vi "Cmd.ReadProgram.vi"(6 "Timeout [ms] (1000)":i32=1000, 8 "error in":errorcluster, 11 "cID in":refnum<k5>) -> (0 "error out":errorcluster, 1 "ProgramNumber":u16, 2 "SDCard":u8, 3 "cID out":refnum<k5>)   [LabVIEW 2016]
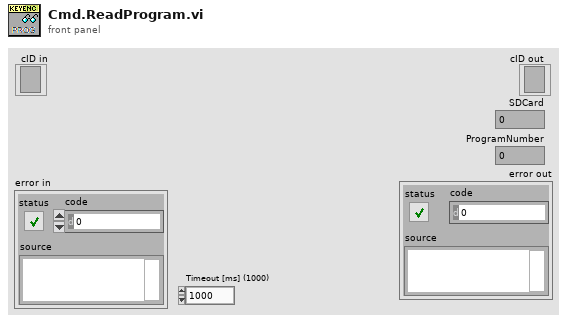
[diagram p1: front panel]
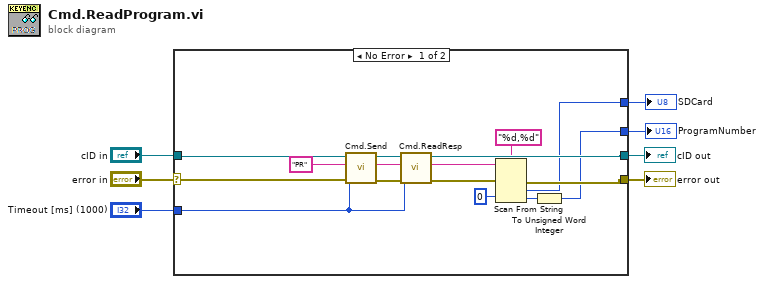
[diagram p0: block diagram]
diagram:
  n1 = case shown="No Error" "error in" {
    selector: "error in" -> [w21 w23]
    tunnel: "Timeout [ms] (1000)" -> [w18 _]
    tunnel: "cID in" -> [w22 w24]
    tunnel: [w17 w24] -> w4
    tunnel: [w12 w23] -> w3
    tunnel: [w11 _] -> w2
    tunnel: [w8 _] -> w1
    frame No Error {
      w9 = u8 0
      w16 = "PR"
      n2 = call "Cmd.Send.vi"("error in (no error)"=w21, "Timeout [ms] (1000)"=w18, "Command"=w16, "connection ID"=w22) -> ("error out"=w19:errorcluster, "connection ID out"=w20:refnum<k5>)  [unwired: 6 in]
      n3 = call "Cmd.ReadResp.vi"("error in (no error)"=w19, "Timeout [ms] (1000)"=w18, "Request"=w16, "connection ID"=w20) -> ("error out"=w13:errorcluster, "ResponseParameters"=w15:string, "connection ID out"=w17:refnum<k5>)  [unwired: 5 in]
      n4 = Scan From String(format string="%d,%d", input string=w15, error in=w13, default 1=w9, default 2=w9) -> (error out=w12:errorcluster, output 1=w11:u8, output 2=w10:u8)  [unwired: 1 in, 2 out]
      n5 = To Unsigned Word Integer(number=w10) -> (unsigned 16bit integer=w8:u16)
    }
    frame Error {
    }
  }
  "cID out" <- w4
  "error out" <- w3
  "SDCard" <- w2
  "ProgramNumber" <- w1
